vi "Set Rx Monitor Properties.vi"(8 "error in":errorcluster, 10 "Rx monitor parameters":T2 {"Strobe" items=["FDX_MON_STROBE_DIS", "FDX_MON_STROBE_STOP", "FDX_MON_STROBE_START"]; "CaptureMode" items=["FDX_MON_SINGLE ", "FDX_MON_CONTINUOUS", "FDX_MON_SELECTIVE", "FDX_MON_RECORDING", "FDX_MON_REROS", "FDX_MON_HMU"]; "DefaultCronoMode" items=["FDX_RX_DEFAULT_ENA_CNT", "FDX_RX_DEFAULT_MON_ENA_ALL", "FDX_RX_DEFAULT_MON_ENA_GOOD"]}, 11 "Rx monitor ref in":T1 format="%.0x") -> (0 "error out":errorcluster, 3 "Rx monitor  ref out":T1 format="%.0x")   [LabVIEW 2020, in "AIM ARINC 664 Scripting.lvlib"]
uses:
  AIM ARINC 664 Scripting.lvlib
  <vilib>/NI VeriStand/Custom Device API/Custom Device API.lvlib
  <vilib>/NI VeriStand/Custom Device API/Set Item Property (U32).vi
  Constants.vi
  <vilib>/NI VeriStand/Custom Device API/Custom Device Item Ref.ctl
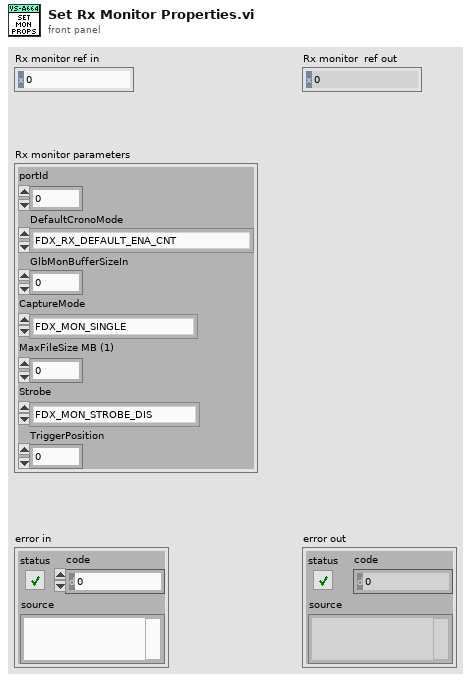
[diagram p1: front panel]
types:
  T1 = typedef "Custom Device API.lvlib/Custom Device Item Ref.ctl" = u64
  T2 = cluster{"portId":u32, "DefaultCronoMode":u32, "GlbMonBufferSizeIn":u32, "CaptureMode":u32, "MaxFileSize MB (1)":u32, "Strobe":u32, "TriggerPosition":u32}
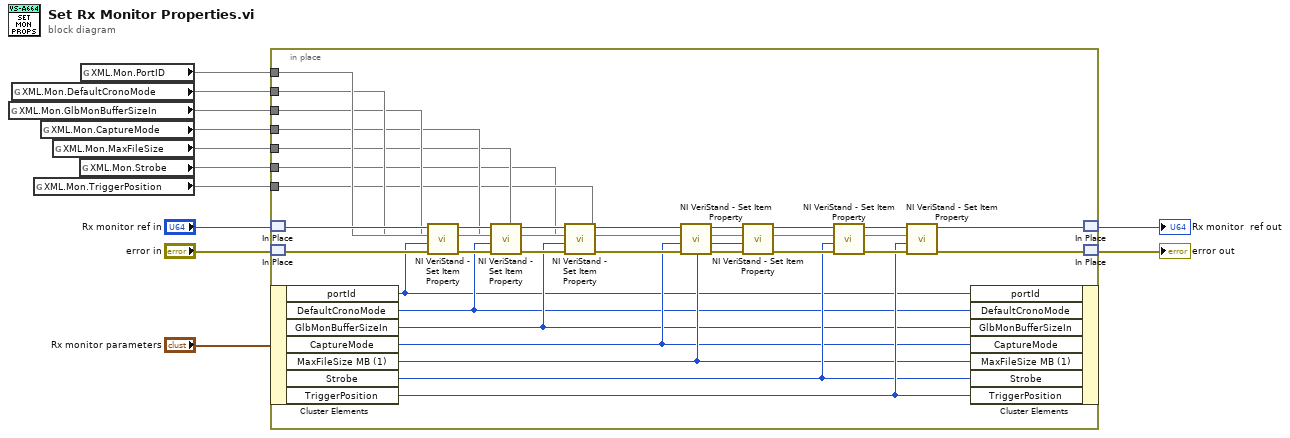
[diagram p0: block diagram]
diagram:
  n1 = global read "Constants.vi" "XML.Mon.GlbMonBufferSizeIn"() -> (w5)
  n2 = global read "Constants.vi" "XML.Mon.DefaultCronoMode"() -> (w6)
  n3 = global read "Constants.vi" "XML.Mon.TriggerPosition"() -> (w2)
  n4 = global read "Constants.vi" "XML.Mon.CaptureMode"() -> (w4)
  n5 = global read "Constants.vi" "XML.Mon.MaxFileSize"() -> (w3)
  n6 = global read "Constants.vi" "XML.Mon.Strobe"() -> (w1)
  n7 = global read "Constants.vi" "XML.Mon.PortID"() -> (w7)
  n8 = in-place {
    in-place-border: w7 -> [w19]
    in-place-border: w6 -> [w18]
    in-place-border: w5 -> [w17]
    in-place-border: w4 -> [w16]
    in-place-border: w3 -> [w15]
    in-place-border: w2 -> [w14]
    in-place-border: w1 -> [w13]
    n9 = in-place-match #1("Rx monitor ref in") -> (w42:T1)
    n10 = in-place-match #2("error in") -> (w35:errorcluster)
    n11 = in-place-cluster #3("Rx monitor parameters") -> ("portId"=w21:u32, "DefaultCronoMode"=w22:u32, "GlbMonBufferSizeIn"=w23:u32, "CaptureMode"=w24:u32, "MaxFileSize MB (1)"=w25:u32, "Strobe"=w26:u32, "TriggerPosition"=w27:u32)
    n12 = call-poly <vilib>:"NI VeriStand - Set Item Property.vi"("error in (no error)"=w35, "Value"=w21, "Property Name"=w19, "Item Ref in"=w42) -> ("error out"=w34:errorcluster, "Item Ref out"=w41:T1)  [unwired: 5 in, 1 out]
    n13 = call-poly <vilib>:"NI VeriStand - Set Item Property.vi"("error in (no error)"=w34, "Value"=w22, "Property Name"=w18, "Item Ref in"=w41) -> ("error out"=w33:errorcluster, "Item Ref out"=w40:T1)  [unwired: 5 in, 1 out]
    n14 = call-poly <vilib>:"NI VeriStand - Set Item Property.vi"("error in (no error)"=w33, "Value"=w23, "Property Name"=w17, "Item Ref in"=w40) -> ("error out"=w32:errorcluster, "Item Ref out"=w39:T1)  [unwired: 5 in, 1 out]
    n15 = call-poly <vilib>:"NI VeriStand - Set Item Property.vi"("error in (no error)"=w32, "Value"=w24, "Property Name"=w16, "Item Ref in"=w39) -> ("error out"=w31:errorcluster, "Item Ref out"=w38:T1)  [unwired: 5 in, 1 out]
    n16 = call-poly <vilib>:"NI VeriStand - Set Item Property.vi"("error in (no error)"=w31, "Value"=w25, "Property Name"=w15, "Item Ref in"=w38) -> ("error out"=w30:errorcluster, "Item Ref out"=w37:T1)  [unwired: 5 in, 1 out]
    n17 = call-poly <vilib>:"NI VeriStand - Set Item Property.vi"("error in (no error)"=w30, "Value"=w26, "Property Name"=w13, "Item Ref in"=w37) -> ("error out"=w29:errorcluster, "Item Ref out"=w36:T1)  [unwired: 5 in, 1 out]
    n18 = call-poly <vilib>:"NI VeriStand - Set Item Property.vi"("error in (no error)"=w29, "Value"=w27, "Property Name"=w14, "Item Ref in"=w36) -> ("error out"=w28:errorcluster, "Item Ref out"=w20:T1)  [unwired: 5 in, 1 out]
    n19 = in-place-cluster #3("portId"=w21, "DefaultCronoMode"=w22, "GlbMonBufferSizeIn"=w23, "CaptureMode"=w24, "MaxFileSize MB (1)"=w25, "Strobe"=w26, "TriggerPosition"=w27) -> ()  [unwired: 1 out]
    n20 = in-place-match #1(w20) -> (→"Rx monitor  ref out":T1)
    n21 = in-place-match #2(w28) -> (→"error out":errorcluster)
  }
